vi "Register Nested Actor.vi"(8 "error in (no error)":errorcluster, 9 "Caller-To-Actor Enqueuer":refnum<class "Message Enqueuer.lvclass">, 10 "Actor UUID":string, 11 "Actor Nest in":refnum<class "Actor Nest.lvclass">) -> (0 "error out":errorcluster, 3 "Actor Nest out":refnum<class "Actor Nest.lvclass">)   [LabVIEW 2018, in "Actor Nest.lvlib" / "Actor Nest.lvclass"]
uses:
  Actor Nest.lvclass
  <vilib>/ActorFramework/Message Enqueuer/Message Enqueuer.lvclass
  Actor Nest.lvclass/Actor Nest.ctl
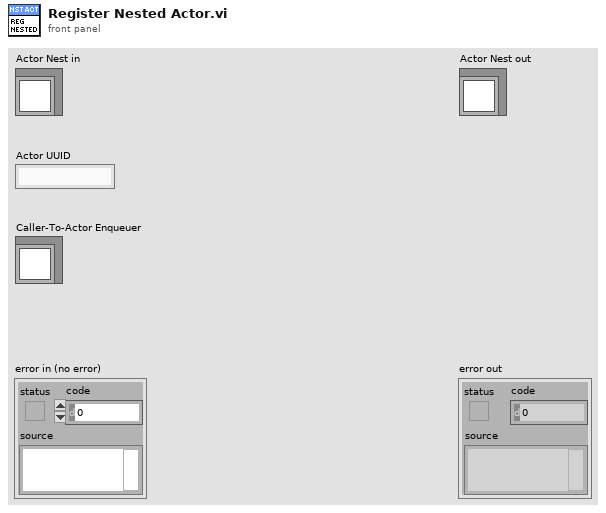
[diagram p1: front panel]
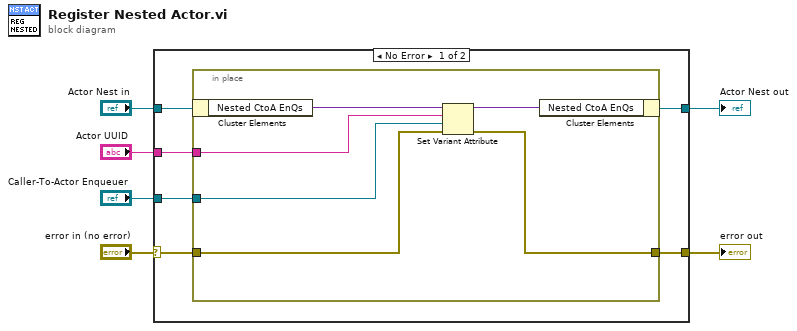
[diagram p0: block diagram]
diagram:
  n1 = case shown="No Error" "error in (no error)" {
    selector: "error in (no error)" -> [w12 w20]
    tunnel: [w9 w20] -> w5
    tunnel: [w10 w19] -> w3
    tunnel: "Actor Nest in" -> [w11 w19]
    tunnel: "Caller-To-Actor Enqueuer" -> [w8 _]
    tunnel: "Actor UUID" -> [w7 _]
    frame No Error {
      n2 = in-place {
        in-place-border: w12 -> [w16]
        in-place-border: [w15] -> w9
        in-place-border: w8 -> [w14]
        in-place-border: w7 -> [w13]
        n3 = in-place-cluster #1(w11) -> ("Nested CtoA EnQs"=w18:variant)
        n4 = Set Variant Attribute(Variant=w18, name=w13, value=w14, error in=w16) -> (Variant out=w17:variant, error out=w15:errorcluster)  [unwired: 1 out]
        n5 = in-place-cluster #1("Nested CtoA EnQs"=w17) -> (w10:refnum<class "Actor Nest.lvclass">)
      }
    }
    frame Error {
    }
  }
  "error out" <- w5
  "Actor Nest out" <- w3
